vi "Test Next Shows Next Test to Run in Flat Test Suite.vi"(8 "error in (no error)":errorcluster, 11 "Test Case In":refnum<class "Test Suite Enumeration Test.lvclass">) -> (0 "error out":errorcluster, 3 "Test Case Out":refnum<class "Test Suite Enumeration Test.lvclass">)   [LabVIEW 2020, in "Test Suite Enumeration Test.lvclass"]
uses:
  Test Suite Enumeration Test.lvclass
  Test Suite Enumeration Test.lvclass/Test Suite Enumeration Test.ctl
  source/API/LUnit Test Suite/LUnit Test Suite.lvclass
  Test Doubles/Test Case Test Double Child/Light Test Case Double.lvclass
  C:/git/astemes-lunit/source/API/LUnit Test Case/LUnit Test Case.lvclass
  C:/git/astemes-lunit/source/Core/Runnable/Runnable.lvclass
  C:/git/astemes-lunit/tests/Test Doubles/Test Case Test Double Child/Light Test Case Double.lvclass
  6b7f3171-a55a-44cc-8f9a-4994299db920.vi
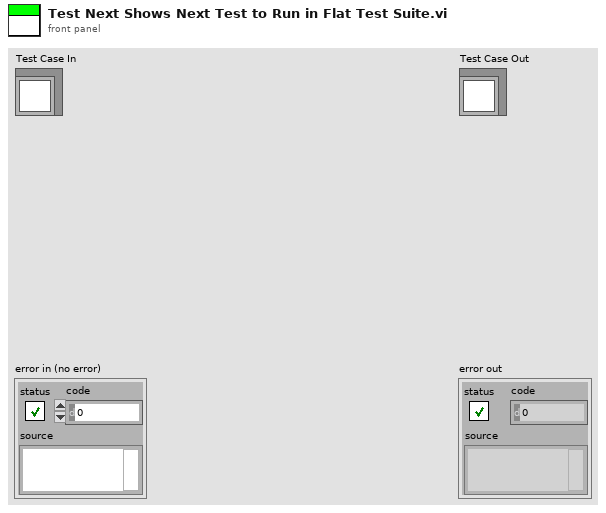
[diagram p1: front panel]
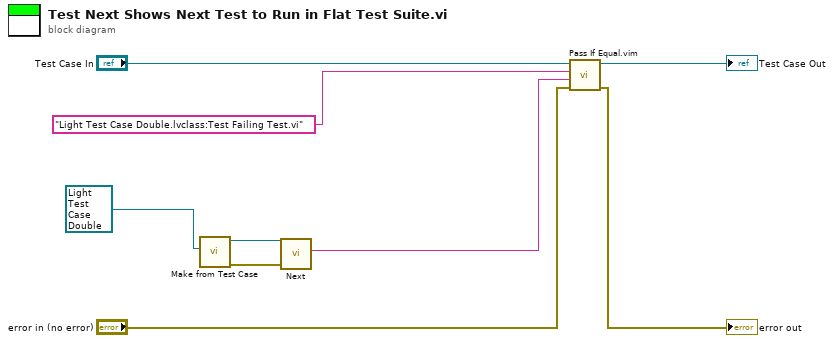
[diagram p0: block diagram]
diagram:
  n1 = call "Make from Test Case.vi"("LUnit Test Case"=refnum<class "Light Test Case Double.lvclass"> refnum ("Light Test Case Double.lvclass")) -> ("error out"=w3:errorcluster, "LUnit Test Suite Out"=w5:refnum<class "LUnit Test Suite.lvclass">)  [unwired: 9 in]
  n2 = call-dynamic "Next.vi"("error in (no error)"=w3, "LUnit Test Suite In"=w5) -> ("Name"=w2:string)  [unwired: 6 in, 3 out]
  n3 = call "Pass If Equal.vim"("error in (no error)"="error in (no error)", "Actual"=w2, "Expected"="Light Test Case Double.lvclass:Test Failing Test.vi" ("Name"), "LUnit Test Case In"="Test Case In") -> ("error out"=→"error out":errorcluster, "LUnit Test Case Out"=→"Test Case Out":refnum<class "Test Suite Enumeration Test.lvclass">)  [unwired: 6 in]
